vi "mlink_ai_scan_status.vi"(8 "error in (no error)":errorcluster, 11 "connection ID":i32=-1) -> (0 "error out":errorcluster, 1 "timestamp":dbl, 2 "busy":bool, 3 "connection ID out":i32)   [LabVIEW 2009, in "MicroDAQ.lvlib" / "mlink.lvlib"]
doc: "This function returns AI scan status and data acquisition start timestamp. If AI scan is started and is waiting for trigger or acquiring data busy is 1, otherwise is 0. If AI scan is started and data is being acquired (trigger occurred or not used) timestamp will contain data acquisition start timestamp. The timestamp contains number of seconds that have elapsed since 00:00:00 Coordinated Universal Time (UTC), Thursday, 1 January 1970. The timestamp returned by function is set to 0 after AI scan initialization function call. If function is called when data \nacquisition is not in progress e.g. trigger not occurred returned, timestamp will equal to 0.\nIn order to convert timestamp value to LabView time value the 2082844800 has to be added to timestamp value."
uses:
  <instrlib>/MicroDAQ/Mlink library wraper/mlink.lvlib
  <instrlib>/MicroDAQ/MLink32.dll
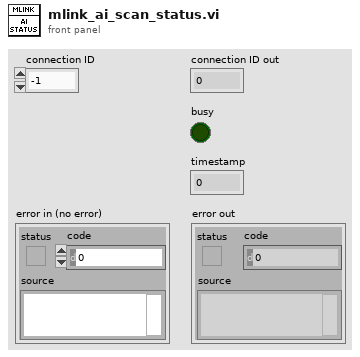
[diagram p1: front panel]
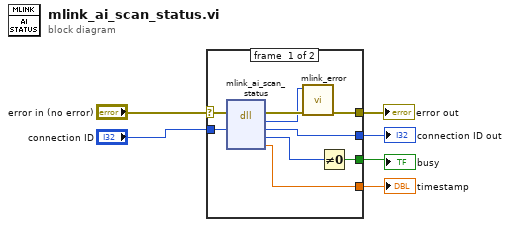
[diagram p0: block diagram]
diagram:
  n1 = case shown="No Error" "error in (no error)" {
    selector: "error in (no error)" -> [w15 w17]
    tunnel: "connection ID" -> [w14 w16]
    tunnel: [w13 w16] -> w4
    tunnel: [w10 w17] -> w3
    tunnel: [w8 _] -> w2
    tunnel: [w7 _] -> w1
    frame #0 {
      n2 = dll-call lib="C:/Program Files (x86)/National Instruments/LabVIEW 2009/instr.lib/MicroDAQ/MLink32.dll" fn="mlink_ai_scan_status" ("MLink64.dll:mlink_dsp_run")(error in=w15, "link_fd"=w14) -> (error out=w12:errorcluster, "return type"=w11:i32, "link_fd"=w13:i32, "busy"=w9:i32, "timestamp"=w7:dbl)  [unwired: 4 in, 1 out]
      n3 = call <instrlib>:"mlink_error.vi"("error in (no error)"=w12, "error code"=w11) -> ("error out"=w10:errorcluster)  [unwired: 9 in]
      n4 = Not Equal To 0?(x=w9) -> (x != 0?=w8:bool)
    }
    frame #1 {
    }
  }
  "connection ID out" <- w4
  "error out" <- w3
  "busy" <- w2
  "timestamp" <- w1
